vi "get status string.vi"(11 "Receive status":string) -> (3 "Status string":string)   [LabVIEW 2014, in "HPCNC.lvlib"]
uses:
  HPCNC.lvlib
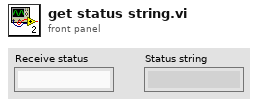
[diagram p1: front panel]
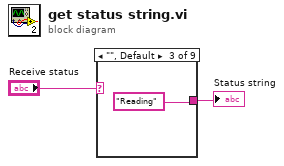
[diagram p0: block diagram]
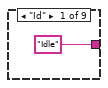
[diagram p2: hidden frame]
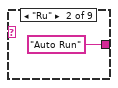
[diagram p3: hidden frame]
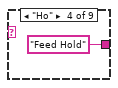
[diagram p4: hidden frame]
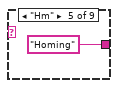
[diagram p5: hidden frame]
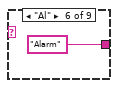
[diagram p6: hidden frame]
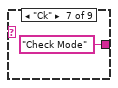
[diagram p7: hidden frame]
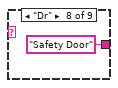
[diagram p8: hidden frame]
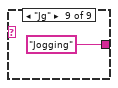
[diagram p9: hidden frame]
diagram:
  n1 = case shown="\"\", Default" "Receive status" {
    tunnel: ["Idle" "Auto Run" "Reading" "Feed Hold" "Homing" "Alarm" "Check Mode" "Safety Door" "Jogging"] -> w2
    frame "Id" {
    }
    frame "Ru" {
    }
    frame "", Default {
    }
    frame "Ho" {
    }
    frame "Hm" {
    }
    frame "Al" {
    }
    frame "Ck" {
    }
    frame "Dr" {
    }
    frame "Jg" {
    }
  }
  "Status string" <- w2
